vi "OpenCreateVI.vi"(8 "error in":errorcluster, 11 "State":T1={"paths"={"index cluster path"=path "C:/Users/bcelis.AMER/Documents/TBDCore/source/Utilities/Cluster to Tag Bus Scripts/Controls/IndexCluster.ctl", "cluster path"=path "C:/Users/bcelis.AMER/Documents/TBDCore/source/Utilities/Cluster to Tag Bus Scripts/Controls/SampleControl.ctl", "cluster to tag bus VI path"=path "C:/Users/bcelis.AMER/Documents/TBDCore/source/Utilities/Cluster to Tag Bus Scripts/ClustertoTagbus.vi", " tag bus to cluster VI path"=path ""}, "write VI ref"=refnum, "read VI ref"=refnum, "base cluster"=variant}) -> (0 "error out":errorcluster, 3 "State out":T1={"paths"={"index cluster path"=path "C:/Users/bcelis.AMER/Documents/TBDCore/source/Utilities/Cluster to Tag Bus Scripts/Controls/IndexCluster.ctl", "cluster path"=path "C:/Users/bcelis.AMER/Documents/TBDCore/source/Utilities/Cluster to Tag Bus Scripts/Controls/SampleControl.ctl", "cluster to tag bus VI path"=path "C:/Users/bcelis.AMER/Documents/TBDCore/source/Utilities/Cluster to Tag Bus Scripts/ClustertoTagbus.vi", " tag bus to cluster VI path"=path ""}, "write VI ref"=refnum, "read VI ref"=refnum, "base cluster"=variant})   [LabVIEW 2013]
uses:
  Controls/StateCluster.ctl
  Controls/PathsCluster.ctl
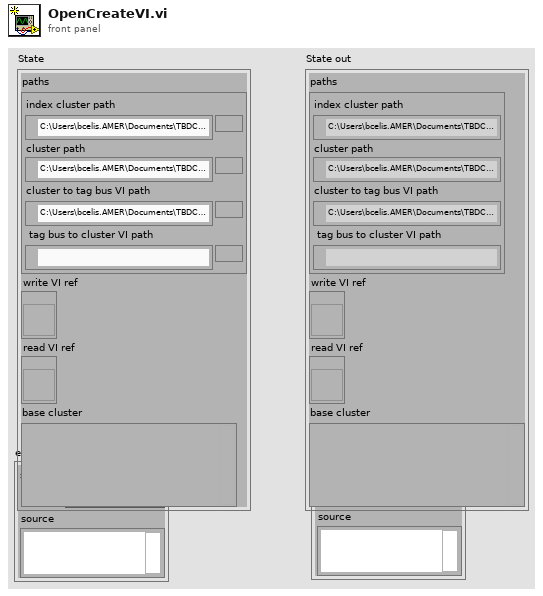
[diagram p1: front panel]
types:
  T1 = typedef "StateCluster.ctl" = cluster{"paths":T2, "write VI ref":refnum<vi>, "read VI ref":refnum<vi>, "base cluster":variant}
  T2 = typedef "PathsCluster.ctl" = cluster{"index cluster path":path, "cluster path":path, "cluster to tag bus VI path":path, " tag bus to cluster VI path":path}
  T3 = enum32{"invalid VI type", "Standard VI", "Control VI", "Global VI", "Polymorphic VI", "Configuration VI", "SubSystem", "Facade VI", "Method VI"}
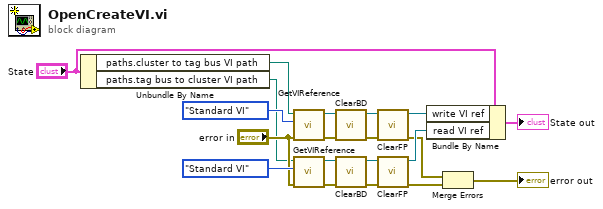
[diagram p0: block diagram]
diagram:
  n1 = Unbundle By Name("State") -> ("paths.cluster to tag bus VI path"=w20:path, "paths.tag bus to cluster VI path"=w5:path)
  n2 = call "GetVIReference.vi"("error in (no error)"="error in", "vi type"=T3."Standard VI", "file path"=w20) -> ("error out"=w18:errorcluster, "reference out"=w16:refnum<vi>)  [unwired: 7 in]
  n3 = call "GetVIReference.vi"("error in (no error)"="error in", "vi type"=T3."Standard VI", "file path"=w5) -> ("error out"=w8:errorcluster, "reference out"=w10:refnum<vi>)  [unwired: 7 in]
  n4 = call "ClearBD.vi"("error in"=w18, "reference"=w16) -> ("error out"=w19:errorcluster, "reference out"=w17:refnum<vi>)  [unwired: 8 in]
  n5 = call "ClearBD.vi"("error in"=w8, "reference"=w10) -> ("error out"=w7:errorcluster, "reference out"=w9:refnum<vi>)  [unwired: 8 in]
  n6 = call "ClearFP.vi"("error in"=w19, "reference"=w17) -> ("error out"=w2:errorcluster, "reference out"=w12:refnum<vi>)  [unwired: 8 in]
  n7 = call "ClearFP.vi"("error in"=w7, "reference"=w9) -> ("error out"=w3:errorcluster, "reference out"=w4:refnum<vi>)  [unwired: 8 in]
  n8 = Bundle By Name(cluster="State", "write VI ref"=w12, "read VI ref"=w4) -> (→"State out":T1)
  n9 = Merge Errors(w2, w3) -> (→"error out":errorcluster)
